vi "Save Single Path.vi"(9 "Path stuff":T10 {"?"."Limits"."StoopidFast (fps)" min=0.0; "?"."Limits"."Jerk (fps^3)" min=0.0 step=1.0; "?"."Limits"."Accel (fps^2)" min=0.0; "?"."Limits"."Velocity (fps)" min=0.0; "?"."Overrides"."Angle Override" step=5.0; "?"."Overrides"."Velocity Override" step=5.0; "?"."Overrides"."Angular Override" step=5.0; "?"."Angular Limits"."Jerk (deg/s^3)" min=0.0 step=1.0; "?"."Angular Limits"."Accel (deg/s^2)" min=0.0; "?"."Angular Limits"."Velocity (deg/s)" min=0.0}, 10 "Filename":string, 11 "Bordeaux paths in":path) -> ()   [LabVIEW 2023]
uses:
  Types/Trajectory Data.ctl
  Types/Segment Type.ctl
  Types/Single Cmd Info.ctl
  <vilib>/picture/picture.llb/imagedata.ctl
  Types/Limits.ctl
  Types/Overrides.ctl
  Types/Angluar Limits.ctl
  Types/Drive Type.ctl
  Types/Path Type.ctl
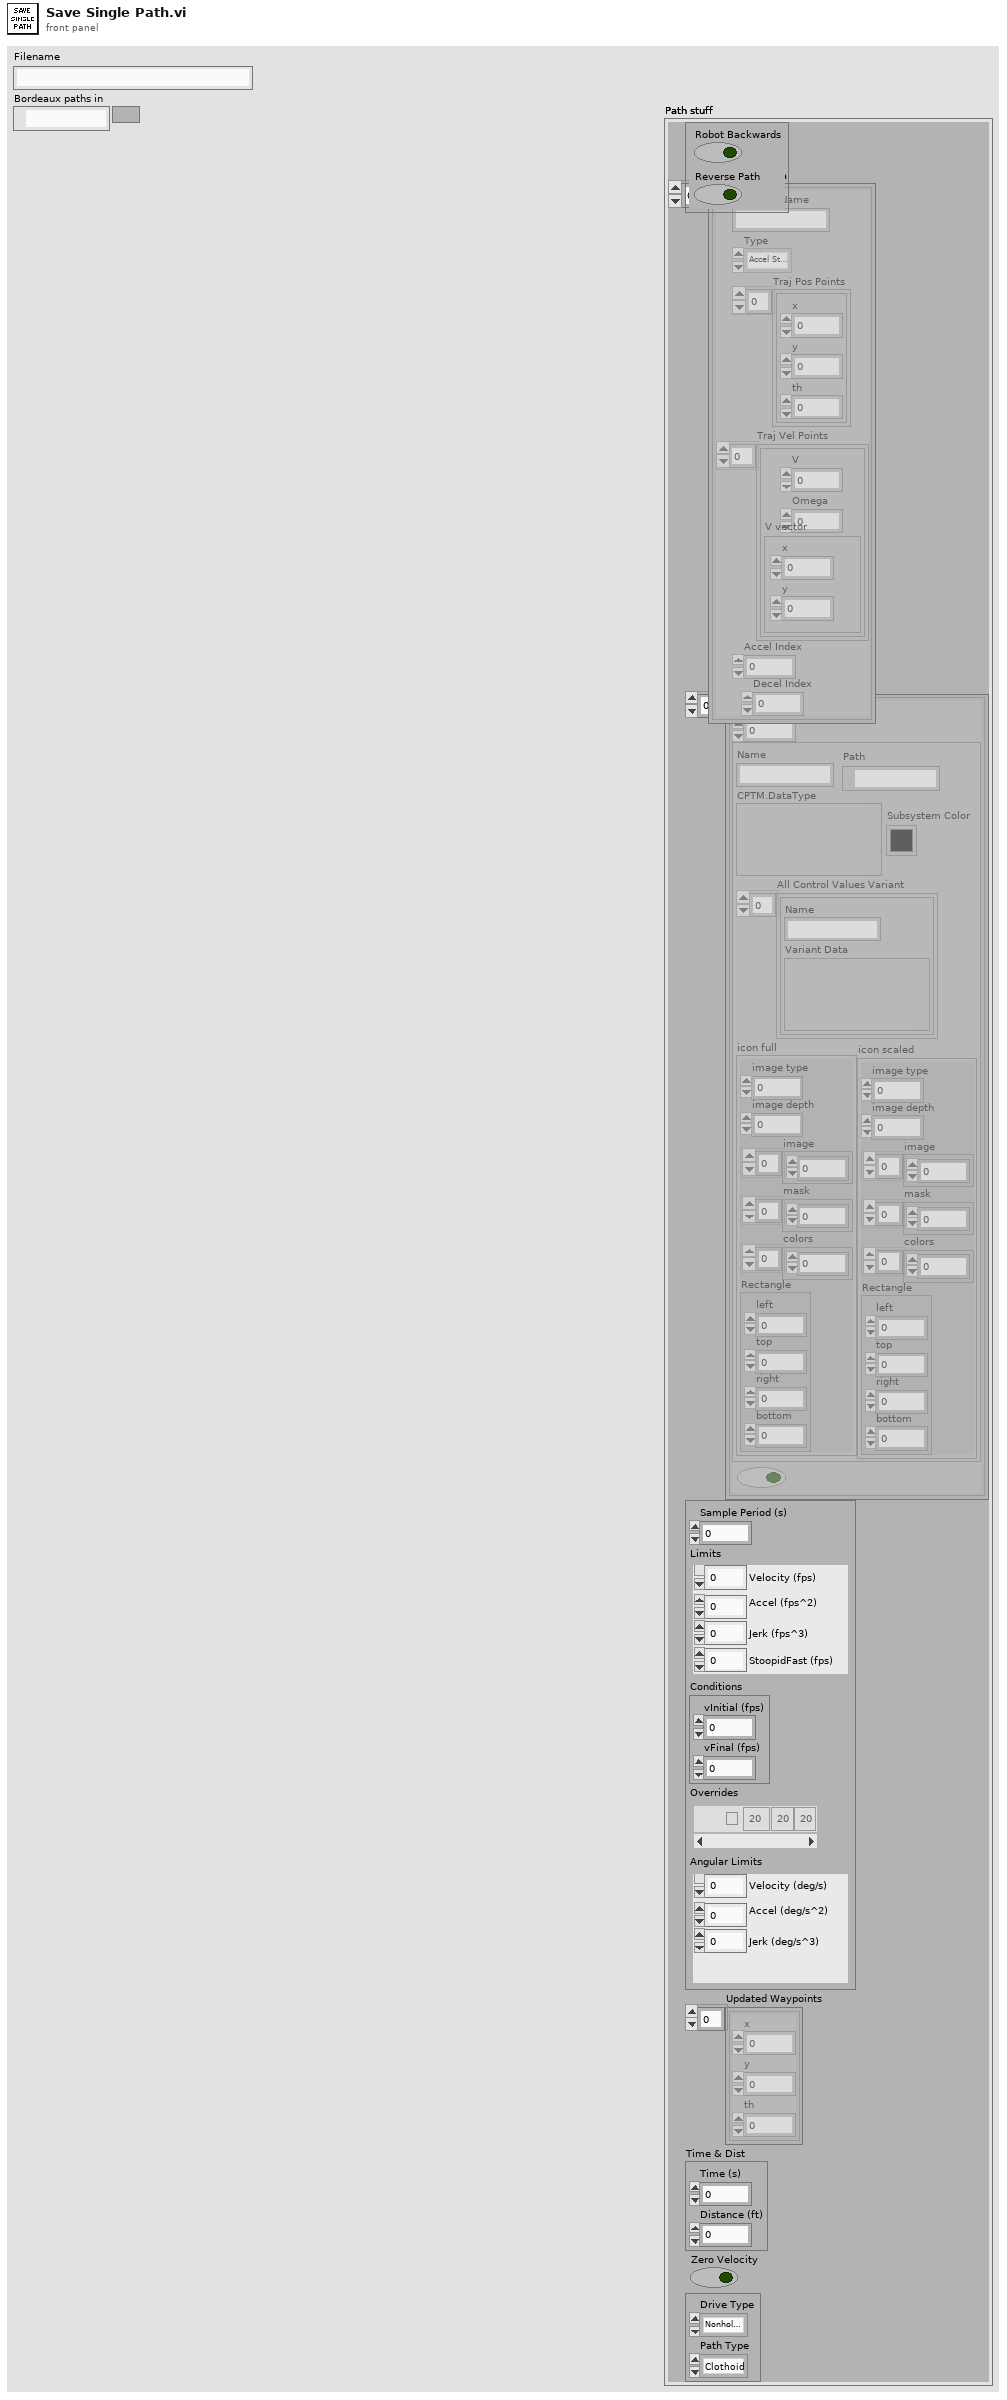
[diagram p1: front panel]
types:
  T1 = typedef "Trajectory Data.ctl" = cluster{"Segment Name":string, "Type":T2, "Traj Pos Points":cluster{"x":dbl, "y":dbl, "th":dbl}[], "Traj Vel Points":cluster{"V":dbl, "Omega":dbl, "V vector":cluster{"y":dbl, "x":dbl}}[], "Accel Index":i32, "Decel Index":i32}[]
  T2 = typedef "Segment Type.ctl" = enum16{"Accel Straight", "Const Straight", "Blend", "Circle", "Bezier"}
  T3 = typedef "Single Cmd Info.ctl" = cluster{"Name":string, "CPTM.DataType":variant, "All Control Values Variant":cluster{"Name":string, "Variant Data":variant}[], "icon full":T4, "icon scaled":T4, "Path":path, "Subsystem Color":u32}
  T4 = typedef "imagedata.ctl" = cluster{"image type":i32, "image depth":i32, "image":u8[], "mask":u8[], "colors":u32[], "Rectangle":cluster{"left":i16, "top":i16, "right":i16, "bottom":i16}}
  T5 = typedef "Limits.ctl" = cluster{"Velocity (fps)":dbl, "Accel (fps^2)":dbl, "Jerk (fps^3)":dbl, "StoopidFast (fps)":dbl}
  T6 = typedef "Overrides.ctl" = cluster{"Count":string, "Angular Override":dbl, "Enabled?":bool, "Velocity Override":dbl, "Angle Override":dbl}[]
  T7 = typedef "Angluar Limits.ctl" = cluster{"Velocity (deg/s)":dbl, "Accel (deg/s^2)":dbl, "Jerk (deg/s^3)":dbl}
  T8 = typedef "Drive Type.ctl" = enum16{"Nonholonomic", "Holonomic"}
  T9 = typedef "Path Type.ctl" = enum16{"Clothoid", "Bezier"}
  T10 = cluster{cluster{"Robot Backwards":bool, "Reverse Path":bool}, "Trajectory Data":T1, "Commands out":cluster{"Time (s)":dbl, T3, bool}[], cluster{"Sample Period (s)":dbl, "Limits":T5, "Conditions":cluster{"vInitial (fps)":dbl, "vFinal (fps)":dbl}, "Overrides":T6, "Angular Limits":T7}, "Updated Waypoints":cluster{"x":dbl, "y":dbl, "th":dbl}[], "Time & Dist":cluster{"Time (s)":dbl, "Distance (ft)":dbl}, "Zero Velocity":bool, cluster{"Drive Type":T8, "Path Type":T9}}
  T11 = cluster{"Robot Backwards":bool, "Reverse Path":bool}
  T12 = cluster{"Sample Period (s)":dbl, "Limits":T5, "Conditions":cluster{"vInitial (fps)":dbl, "vFinal (fps)":dbl}, "Overrides":T6, "Angular Limits":T7}
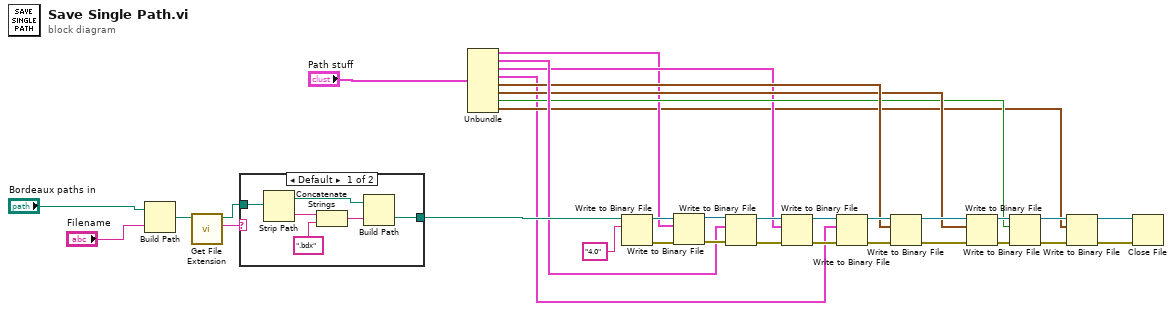
[diagram p0: block diagram]
diagram:
  n1 = Build Path(base path="Bordeaux paths in", name or relative path="Filename") -> (appended path=w31:path)
  n2 = call <vilib>:"Get File Extension.vi"("file"=w31) -> ("lowercase file extension"=w32:string, "dup file"=w33:path)  [unwired: 6 in, 3 out]
  n3 = case shown="Default" w32 {
    tunnel: w33 -> [w39 w41]
    tunnel: [w36 w41] -> w34
    frame Default {
      n4 = Strip Path(path=w39) -> (stripped path=w37:path, name=w38:string)
      n5 = Concatenate Strings(w38, ".bdx") -> (w35:string)
      n6 = Build Path(base path=w37, name or relative path=w35) -> (appended path=w36:path)
    }
    frame "bdx" {
    }
  }
  n7 = Unbundle("Path stuff") -> (w6:T11, "Trajectory Data"=w11:T1, "Commands out"=w7:cluster{"Time (s)":dbl, T3, bool}[], w2:T12, "Updated Waypoints"=w10:cluster{"x":dbl, "y":dbl, "th":dbl}[], "Time & Dist"=w9:cluster{"Time (s)":dbl, "Distance (ft)":dbl}, "Zero Velocity"=w8:bool, w3:cluster{"Drive Type":T8, "Path Type":T9})
  n8 = Write to Binary File(file (use dialog)=w34, data="4.0") -> (refnum out=w14:refnum<file>, error out=w20:errorcluster)  [unwired: 4 in, 1 out]
  n9 = Write to Binary File(file (use dialog)=w14, data=w6, error in=w20) -> (refnum out=w16:refnum<file>, error out=w21:errorcluster)  [unwired: 3 in, 1 out]
  n10 = Write to Binary File(file (use dialog)=w16, data=w11, error in=w21) -> (refnum out=w17:refnum<file>, error out=w22:errorcluster)  [unwired: 3 in, 1 out]
  n11 = Write to Binary File(file (use dialog)=w17, data=w7, error in=w22) -> (refnum out=w18:refnum<file>, error out=w23:errorcluster)  [unwired: 3 in, 1 out]
  n12 = Write to Binary File(file (use dialog)=w18, data=w2, error in=w23) -> (refnum out=w12:refnum<file>, error out=w24:errorcluster)  [unwired: 3 in, 1 out]
  n13 = Write to Binary File(file (use dialog)=w12, data=w10, error in=w24) -> (refnum out=w15:refnum<file>, error out=w25:errorcluster)  [unwired: 3 in, 1 out]
  n14 = Write to Binary File(file (use dialog)=w15, data=w9, error in=w25) -> (refnum out=w19:refnum<file>, error out=w26:errorcluster)  [unwired: 3 in, 1 out]
  n15 = Write to Binary File(file (use dialog)=w19, data=w8, error in=w26) -> (refnum out=w5:refnum<file>, error out=w4:errorcluster)  [unwired: 3 in, 1 out]
  n16 = Write to Binary File(file (use dialog)=w5, data=w3, error in=w4) -> (refnum out=w28:refnum<file>, error out=w27:errorcluster)  [unwired: 3 in, 1 out]
  n17 = Close File(refnum=w28, error in=w27) -> ()  [unwired: 2 out]
